vi "Get Weight.vi"(8 "error in (no error)":errorcluster, 9 "Channel":i32, 10 "Bias Voltage (V)":dbl, 11 "Example in":refnum<class "Instrument.LN2.lvclass">) -> (0 "error out":errorcluster, 3 "Example out":refnum<class "Instrument.LN2.lvclass">)   [LabVIEW 2019, in "Instrument.LN2.lvclass"]
uses:
  Instrument.LN2.lvclass
  C:/Program Files (x86)/National Instruments/LabVIEW 2019/user.lib/LevyLab/Instrument Framework/SMOs/Instrument/Instrument.lvclass
  Typedefs/Instrument.LN2.Commands--Enum.ctl
  <userlib>/LevyLab/Instrument Framework/SMOs/Instrument/Instrument.lvclass/Instrument.ctl
  67792bfe-8e2c-4879-abc2-cb448bcec168.vi
  67792bfe-8e2c-4879-abc2-cb448bcec168.vi/b27858a4-9378-45b3-ad98-96f8064b6f97.vi
  <userlib>/LevyLab/Instrument Framework/SMOs/Instrument/API/Send and Receive.vi
  67792bfe-8e2c-4879-abc2-cb448bcec168.vi/7fb27a88-14d0-419e-b870-207e27305ca3.vi
  <userlib>/LevyLab/Instrument Framework/SMOs/Instrument/Private/Get Client Type.vi
  67792bfe-8e2c-4879-abc2-cb448bcec168.vi/b27858a4-9378-45b3-ad98-96f8064b6f97.vi/0f9c8e3a-82ca-4f6b-b951-734d00e7f4a3.vi
  67792bfe-8e2c-4879-abc2-cb448bcec168.vi/b27858a4-9378-45b3-ad98-96f8064b6f97.vi/744578d7-8aca-4707-bf09-f9f3826c2f84.vi
  67792bfe-8e2c-4879-abc2-cb448bcec168.vi/7fb27a88-14d0-419e-b870-207e27305ca3.vi/814d012b-71ba-45f0-9e1d-83865a8d36f1.vi
  67792bfe-8e2c-4879-abc2-cb448bcec168.vi/7fb27a88-14d0-419e-b870-207e27305ca3.vi/7ddf0c15-3fb4-4a01-bf70-ab981701f6af.vi
  67792bfe-8e2c-4879-abc2-cb448bcec168.vi/7fb27a88-14d0-419e-b870-207e27305ca3.vi/814d012b-71ba-45f0-9e1d-83865a8d36f1.vi/42192020-c11b-422f-8558-60e557ac31ea.vi
  67792bfe-8e2c-4879-abc2-cb448bcec168.vi/7fb27a88-14d0-419e-b870-207e27305ca3.vi/814d012b-71ba-45f0-9e1d-83865a8d36f1.vi/7e55447b-afb4-47dd-b1a0-4cf249da81e6.vi
  <userlib>/LevyLab/Instrument Framework/SMOs/Instrument/Private/Get RC Connection Status.vi
  <userlib>/LevyLab/Instrument Framework/SMOs/Instrument/API/Enum to String.vi
  <userlib>/LevyLab/Instrument Framework/SMOs/RemoteControl/API/Send and Receive.vi
  <vilib>/Utility/Data Type/Get Type Information.vi
  <vilib>/JDP Science/JSONtext/JSON text to Variant.vi
  <userlib>/LevyLab/Instrument Framework/SMOs/Instrument/API/Instrument.GetPublicEvents.vi
  <vilib>/JDP Science/JSONtext/Variant to JSON Text.vi
  <vilib>/National Instruments/GUID Generator/Guid Generator.vi
  <userlib>/LevyLab/Instrument Framework/SMOs/Instrument/API/Instrument.MessageToProcess.vi
  <userlib>/LevyLab/Instrument Framework/SMOs/Instrument/Private/Instrument.MessageFromProcess.EventStructure.vi
  <vilib>/JDP Science/JSONtext/LVClass Serializer/JSONtext LVClass Serializer.lvclass
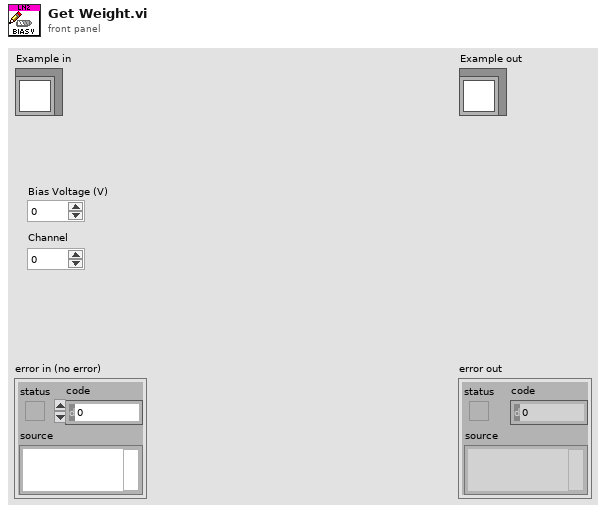
[diagram p1: front panel]
types:
  T1 = typedef "Instrument.LN2.lvclass/Instrument.LN2.Commands--Enum.ctl" = enum16{"command0", "command1", "command2"}
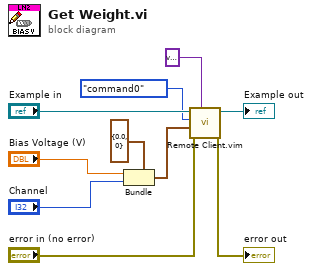
[diagram p0: block diagram]
diagram:
  n1 = Bundle(cluster=cluster{"Bias Voltage (V)":dbl, "Channel":i32} {"Bias Voltage (V)"=0.0, "Channel"=0} ("output cluster"), "Bias Voltage (V)"="Bias Voltage (V)", "Channel"="Channel") -> (w3:cluster{"Bias Voltage (V)":dbl, "Channel":i32})
  n2 = call "Remote Client.vim"("Data Out type"=variant, "error in (no error)"="error in (no error)", "params"=w3, "method"=Instrument.LN2.Commands--Enum."command0" ("Commands"), "Instrument in"="Example in") -> ("error out"=→"error out":errorcluster, "Instrument out"=→"Example out":refnum<class "Instrument.LN2.lvclass">)  [unwired: 3 in, 2 out]
